vi "Clone.vi"(8 "Error In":errorcluster, 11 "reference in":refnum<class "Circle.lvclass">) -> (0 "Error Out":errorcluster, 2 "Return(LabVIEW Object)":refnum<class "ICloneable.lvclass">, 3 "reference out":refnum<class "Circle.lvclass">)   [LabVIEW 2020, in "Circle.lvclass"]
uses:
  Circle.lvclass
  C:/Projects/DesignPatterns/PrototypePattern/ICloneable_interface/ICloneable.lvclass
  ICloneable_interface/ICloneable.lvclass
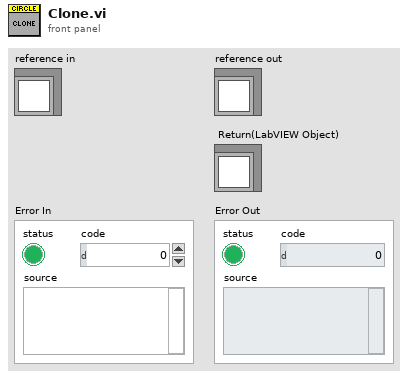
[diagram p1: front panel]
types:
  T1 = typedef "Circle.lvclass/ObjectAttributes.ctl" = cluster{"_radius":i32}
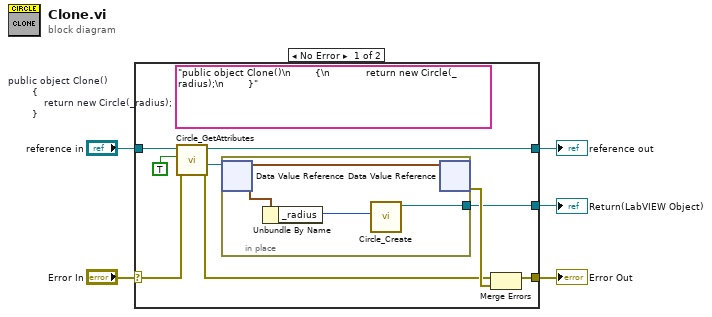
[diagram p0: block diagram]
diagram:
  n1 = case shown="No Error" "Error In" {
    selector: "Error In" -> [w13 w19]
    tunnel: [w10 w19] -> w4
    tunnel: [w11 w18] -> w2
    tunnel: "reference in" -> [w14 w18]
    tunnel: [w6 _] -> w1
    frame No Error {
      (unwired) "public object Clone()\n        {\n            return new Circle(_radius);\n        }"  # public object Clone()         {             return new Circle(_radius);         }
      n2 = call "Circle_GetAttributes.vi"("error in (no error)"=w13, "OnlyGetDvrReference(False)"=TRUE, "reference in"=w14) -> ("error out"=w8:errorcluster, "DataRef"=w9:refnum<data-value>, "reference out"=w11:refnum<class "Circle.lvclass">)  [unwired: 5 in, 1 out]
      n3 = in-place {
        in-place-border: [w15] -> w6
        n4 = in-place-dvr #1(w9) -> (w17:T1)  [unwired: 1 out]
        n5 = Unbundle By Name(w17) -> ("_radius"=w16:i32)
        n6 = call "Circle_Create.vi"("R"=w16) -> ("reference out"=w15:refnum<class "Circle.lvclass">)  [unwired: 9 in, 1 out]
        n7 = in-place-dvr #1(w17) -> (w12:errorcluster)  [unwired: 1 out]
      }
      n8 = Merge Errors(w8, w12) -> (w10:errorcluster)
    }
    frame Error {
    }
  }
  "Error Out" <- w4
  "reference out" <- w2
  "Return(LabVIEW Object)" <- w1
